vi "GPIO Write.vi"(9 "PinValue":u32, 10 "PinMask":u32, 11 "DevIndex":i32) -> (3 "function return":i32)   [LabVIEW 2010, in "usb2gpio.lvlib"]
doc: "int WINAPI GPIO_Write(int DevIndex,unsigned int PinMask, unsigned int PinValue);"
uses:
  usb2gpio.lvlib
  USB2XXX.dll
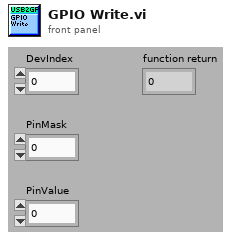
[diagram p1: front panel]
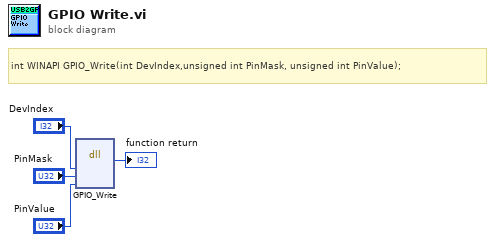
[diagram p0: block diagram]
diagram:
  # "int WINAPI GPIO_Write(int DevIndex,unsigned int PinMask, unsigned int PinValue);"
  n1 = dll-call lib="G:/OtherWork/USB2XXX_Example/trunk/Labview/PublicFiles/usb2gpio/USB2XXX.*" fn="GPIO_Write"("DevIndex"="DevIndex", "PinMask"="PinMask", "PinValue"="PinValue") -> (→"function return":i32)  [unwired: 6 in, 2 out]
